vi "Perform_AFP.vi"(7 "AFP Efficiency":dbl, 8 "AFP Target":i32, 9 "rho-":dbl[](array[numeric]), 10 "rho0":dbl[](array[numeric]), 11 "rho+":dbl[](array[numeric])) -> (1 "rho- out":dbl[](array[numeric]), 2 "rho0 out":dbl[](array[numeric]), 3 "rho+ out":dbl[](array[numeric]))   [LabVIEW 2018]
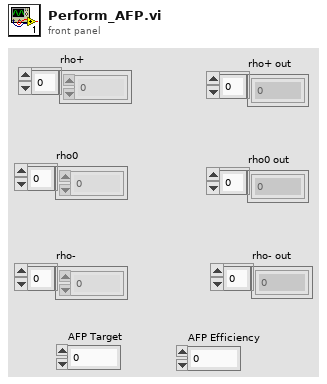
[diagram p1: front panel]
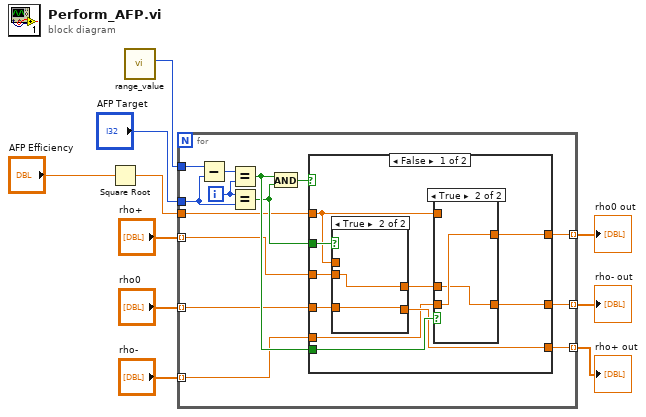
[diagram p0: block diagram]
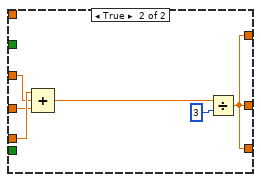
[diagram p4: hidden frame]
diagram:
  n1 = Square Root(x="AFP Efficiency") -> (sqrt(x)=w1:dbl)
  n2 = call "range_value.vi"() -> ("NumBins"=w3:i32)  [unwired: 10 in, 1 out]
  n3 = for {
    tunnel: "rho+" -> [w17] mode=indexing
    tunnel: "rho0" -> [w16] mode=indexing
    tunnel: "rho-" -> [w15] mode=indexing
    tunnel: w3 -> [w24]
    tunnel: "AFP Target" -> [w21]
    tunnel: [w14] -> w6 mode=indexing
    tunnel: [w13] -> w5 mode=indexing
    tunnel: [w12] -> w4 mode=indexing
    tunnel: w1 -> [w11]
    i -> [w22]
    n4 = Subtract(x=w24, y=w21) -> (x-y=w23:i32)
    n5 = Equal?(x=w23, y=w22) -> (x = y?=w20:bool)
    n6 = Equal?(x=w22, y=w21) -> (x = y?=w18:bool)
    n7 = And(x=w20, y=w18) -> (x .and. y?=w19:bool)
    n8 = case shown="False" w19 {
      tunnel: w20 -> [w34 _]
      tunnel: w18 -> [w33 _]
      tunnel: w17 -> [w32 w47]
      tunnel: w16 -> [w31 w46]
      tunnel: [w29 w43] -> w14
      tunnel: w15 -> [w28 w48]
      tunnel: [w27 w43] -> w12
      tunnel: [w26 w43] -> w13
      tunnel: w11 -> [w25 _]
      frame False {
        n9 = case shown="True" w33 {
          tunnel: w32 -> [w36 w38]
          tunnel: w31 -> [w35 w37]
          tunnel: [w36 w37] -> w29
          tunnel: [w35 w38] -> w30
          tunnel: w25 -> [_ _]
          frame False {
          }
          frame True {
          }
        }
        n10 = case shown="True" w34 {
          tunnel: w30 -> [w40 w41]
          tunnel: [w40 w42] -> w26
          tunnel: w28 -> [w39 w42]
          tunnel: [w39 w41] -> w27
          tunnel: w25 -> [_ _]
          frame False {
          }
          frame True {
          }
        }
      }
      frame True {
        n11 = Compound Arithmetic op=ADD(w48, w47, w46) -> (w45:dbl)
        n12 = Divide(x=w45, y=3) -> (x/y=w43:dbl)
      }
    }
  }
  "rho+ out" <- w6
  "rho0 out" <- w5
  "rho- out" <- w4
